vi "Ctor.vi"(8 "error in (no error)":errorcluster, 9 "Value (None)":string, 10 "Name (None)":string, 11 "Type":T1) -> (0 "error out":errorcluster, 3 "NodeRef":refnum<data-value>)   [LabVIEW 2020, in "PicoG-ParserLexer.lvlib" / "Node.lvclass"]
doc: "Instantiates the node with the given properties.\n\n<b>Name</b>: The keyword, variable name, instruction name, type name, etc. Name will be empty for argument literals.\n\n<b>Value</b>: Either the default value for a type definition or an instruction argument literal. Will be emtpy for nodes that are not default values or argument literals.\n\n<b>Error Codes:</b>\n<b>1</b>: Invalid <b>Value</b> provided for the given <b>Type</b>."
uses:
  Node.lvclass
  AST Node Type.ctl
  PicoG-ParserLexer.lvlib
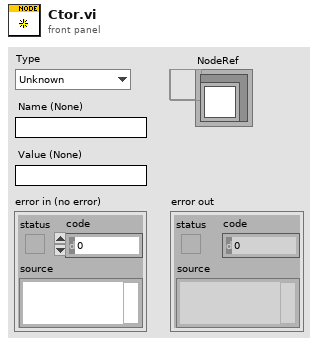
[diagram p1: front panel]
types:
  T1 = typedef "PicoG-ParserLexer.lvlib/AST Node Type.ctl" = enum16{"Unknown", "Keyword", "Array", "Cluster", "Numeric", "Boolean", "String", "Identifier"}
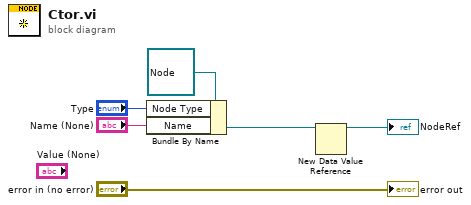
[diagram p0: block diagram]
diagram:
  n1 = Bundle By Name(cluster=refnum<class "Node.lvclass"> refnum ("PicoG-ParserLexer:Node.lvclass"), "Node Type"="Type", "Name"="Name (None)") -> (w2:refnum<class "Node.lvclass">)
  n2 = New Data Value Reference(data value=w2) -> (data value reference=→"NodeRef":refnum<data-value>)  [unwired: 1 in, 1 out]
  "error out" <- "error in (no error)"
